vi "SetTickTime.vi"(8 "Uart Input":cluster{u64} {"?" format="%x"}, 10 "Tick Interval (ms)":u32=50, 11 "Error Input":errorcluster) -> (0 "Uart Output":cluster{u64} {"?" format="%x"}, 3 "Error Output":errorcluster)   [LabVIEW 2019]
doc: "Set <B>Tick Interval</B> of the <B>On Tick</B> event."
uses:
  dll/LabViewUart.dll
panel:
  # "Set Tick Interval"
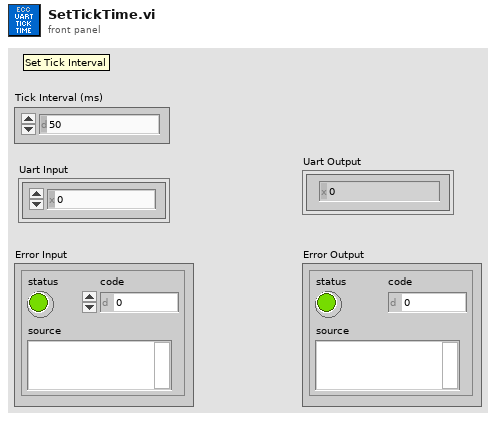
[diagram p1: front panel]
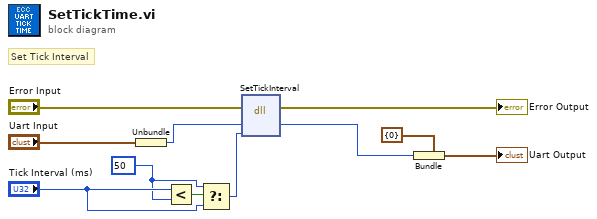
[diagram p0: block diagram]
diagram:
  w2 = u32 50 ("y")
  # "Set Tick Interval"
  n1 = Unbundle("Uart Input") -> (w4:u64)
  n2 = Less?(x="Tick Interval (ms)", y=w2) -> (x < y?=w5:bool)
  n3 = Select(t=w2, s=w5, f="Tick Interval (ms)") -> (s? t:f=w1:u32)
  n4 = dll-call lib="D:/Google Drive/INC-2020/INC352/INC352-2020/LabVIEW/examples/uart-cmdex/SubVI/dll/LabViewUart.dll" fn="SetTickInterval"(error in="Error Input", "Uart Handle"=w4, "Tick Interval"=w1) -> (error out=→"Error Output":errorcluster, "Uart Handle"=w7:u64)  [unwired: 4 in, 1 out]
  n5 = Bundle(cluster=cluster{u64} {0}, w7) -> (→"Uart Output":cluster{u64})
